vi "startIVSweepAndWait.vi"(8 "error in (no error)":errorcluster, 10 "Configure Sweep 2":T1, 11 "Instrument.LockinAPI in":refnum<class "Instrument.LockinAPI.lvclass">) -> (0 "error out":errorcluster, 3 "Instrument.LockinAPI out":refnum<class "Instrument.LockinAPI.lvclass">)   [LabVIEW 2019, in "Instrument.LockinAPI.lvclass"]
uses:
  Instrument.LockinAPI.lvclass
  Typedefs/LockinAPI.SweepConfig--Cluster.ctl
  Typedefs/LockinAPI.SweepChannel--Cluster.ctl
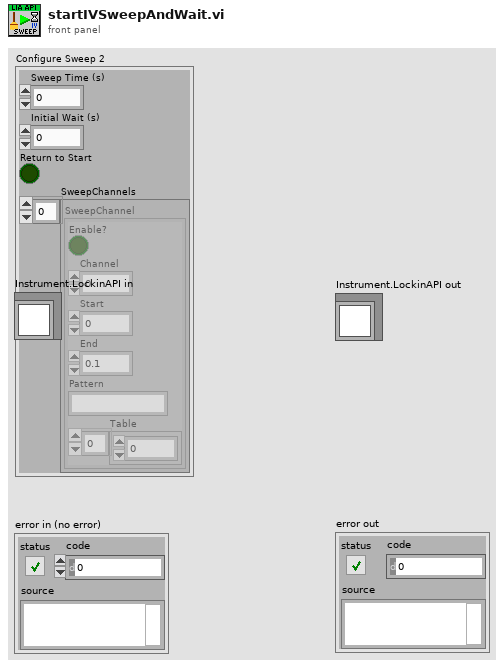
[diagram p1: front panel]
types:
  T1 = typedef "Instrument.LockinAPI.lvclass/LockinAPI.SweepConfig--Cluster.ctl" = cluster{"Sweep Time (s)":dbl, "Initial Wait (s)":dbl, "Return to Start":bool, "SweepChannels":T2[]}
  T2 = typedef "Instrument.LockinAPI.lvclass/LockinAPI.SweepChannel--Cluster.ctl" = cluster{"Enable?":bool, "Channel":u16, "Start":dbl, "End":dbl, "Pattern":string, "Table":dbl[]}
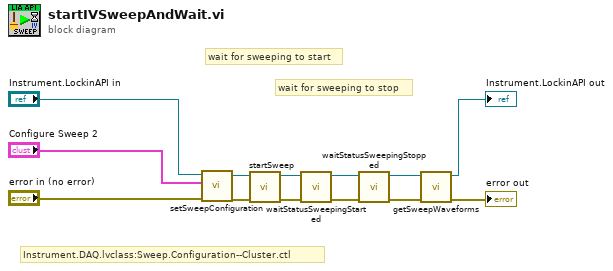
[diagram p0: block diagram]
diagram:
  # "Instrument.DAQ.lvclass:Sweep.Configuration--Cluster.ctl"
  # "wait for sweeping to stop"
  # "wait for sweeping to start"
  n1 = call-dynamic "setSweepConfiguration.vi"("error in (no error)"="error in (no error)", "SweepConfiguration"="Configure Sweep 2", "Instrument.LockinAPI in"="Instrument.LockinAPI in") -> ("error out"=w9:errorcluster, "Instrument.LockinAPI out"=w10:refnum<class "Instrument.LockinAPI.lvclass">)  [unwired: 7 in]
  n2 = call-dynamic "startSweep.vi"("error in (no error)"=w9, "Instrument.LockinAPI in"=w10) -> ("error out"=w5:errorcluster, "Instrument.LockinAPI out"=w6:refnum<class "Instrument.LockinAPI.lvclass">)  [unwired: 8 in]
  n3 = call-dynamic "waitStatusSweepingStarted.vi"("error in (no error)"=w5, "Instrument.LockinAPI in"=w6) -> ("error out"=w4:errorcluster, "Instrument.LockinAPI out"=w7:refnum<class "Instrument.LockinAPI.lvclass">)  [unwired: 8 in]
  n4 = call-dynamic "waitStatusSweepingStopped.vi"("error in (no error)"=w4, "Instrument.LockinAPI in"=w7) -> ("error out"=w3:errorcluster, "Instrument.LockinAPI out"=w2:refnum<class "Instrument.LockinAPI.lvclass">)  [unwired: 8 in]
  n5 = call-dynamic "getSweepWaveforms.vi"("error in (no error)"=w3, "Instrument.LockinAPI in"=w2) -> ("error out"=→"error out":errorcluster, "Instrument.LockinAPI out"=→"Instrument.LockinAPI out":refnum<class "Instrument.LockinAPI.lvclass">)  [unwired: 6 in, 2 out]
